vi "ni579x Validate LO Scope.vi"(0 "Register Bus":T1, 1 "scope":string, 11 "Error In":errorcluster) -> (4 "Register Bus (out)":T1, 15 "Error Out":errorcluster)   [LabVIEW 2015, in "ni579x Config v2 Host.lvlib"]
uses:
  <instrlib>/ni579x/Config/v2/Host/ni579x Config v2 Host.lvlib
  <instrlib>/_niInstr/Register Bus/v0/Host/Public/Register Bus Session.ctl
  <instrlib>/_niInstr/Register Bus/v0/Host/Private/Session Data.ctl
  <instrlib>/_niInstr/Register Bus/v0/Host/niInstr Register Bus v0 Host.lvlib
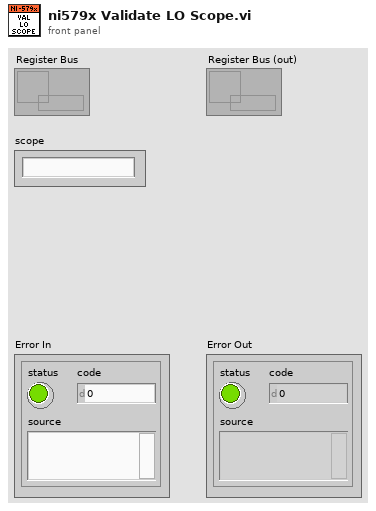
[diagram p1: front panel]
types:
  T1 = typedef "niInstr Register Bus v0 Host.lvlib/Register Bus Session.ctl" = refnum<queue>
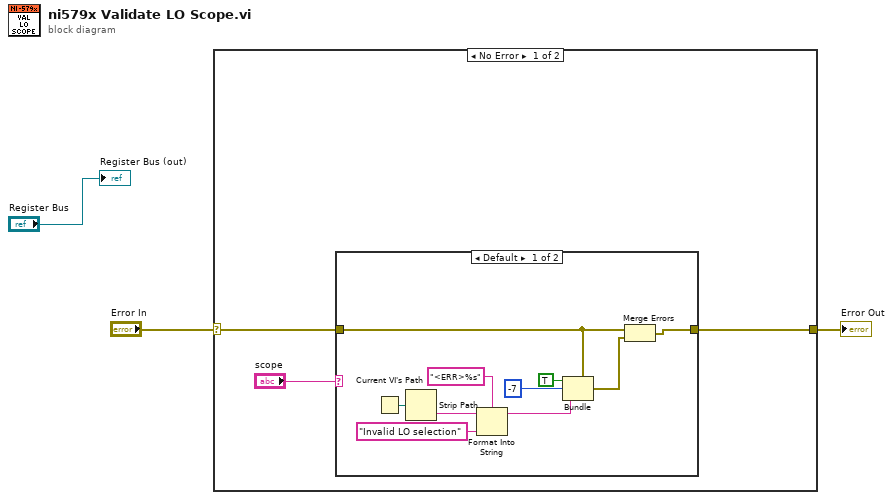
[diagram p0: block diagram]
diagram:
  n1 = case shown="No Error" "Error In" {
    selector: "Error In" -> [w4 w18]
    tunnel: [w5 w18] -> w2
    frame No Error {
      n2 = case shown="Default" "scope" {
        tunnel: w4 -> [w9 w17]
        tunnel: [w7 w17] -> w5
        frame Default {
          n3 = Current VI's Path() -> (path=w11:path)
          n4 = Strip Path(path=w11) -> (name=w12:string)  [unwired: 1 out]
          n5 = Format Into String(format string="<ERR>%s", initial string=w12, "Invalid LO selection" ("input 1")) -> (resulting string=w13:string)  [unwired: 1 in, 1 out]
          n6 = Bundle(cluster=w9, "status"=TRUE, "code"=-7, "source"=w13) -> (w8:errorcluster)
          n7 = Merge Errors(w9, w8) -> (w7:errorcluster)
        }
        frame "LO1", "LO2" {
        }
      }
    }
    frame Error {
    }
  }
  "Error Out" <- w2
  "Register Bus (out)" <- "Register Bus"
